vi "Programmingapplication_429B.vi"() -> (0 "command line":string=" -openD:\\20161122\\LNK01E-213300ALF\\LNK213-300ALF\\SW0077076V1-04.hex", 3 "Result":bool)   [LabVIEW 2011]
panel:
  out "text":string
  out "match + rest of string":string
  out "standard output":string
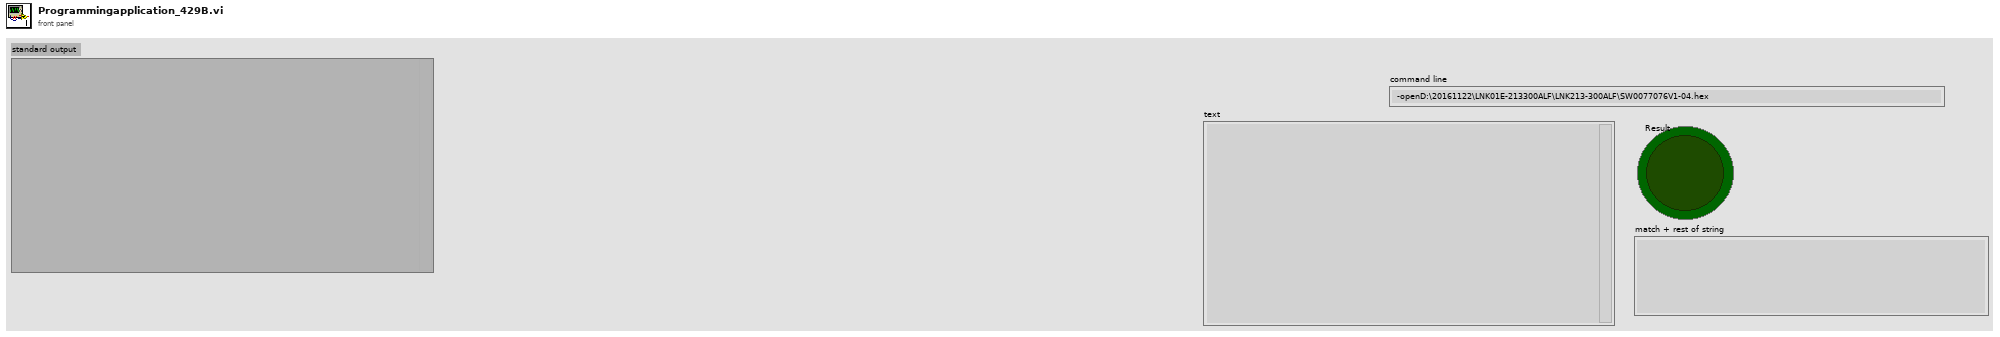
[diagram p1: front panel]
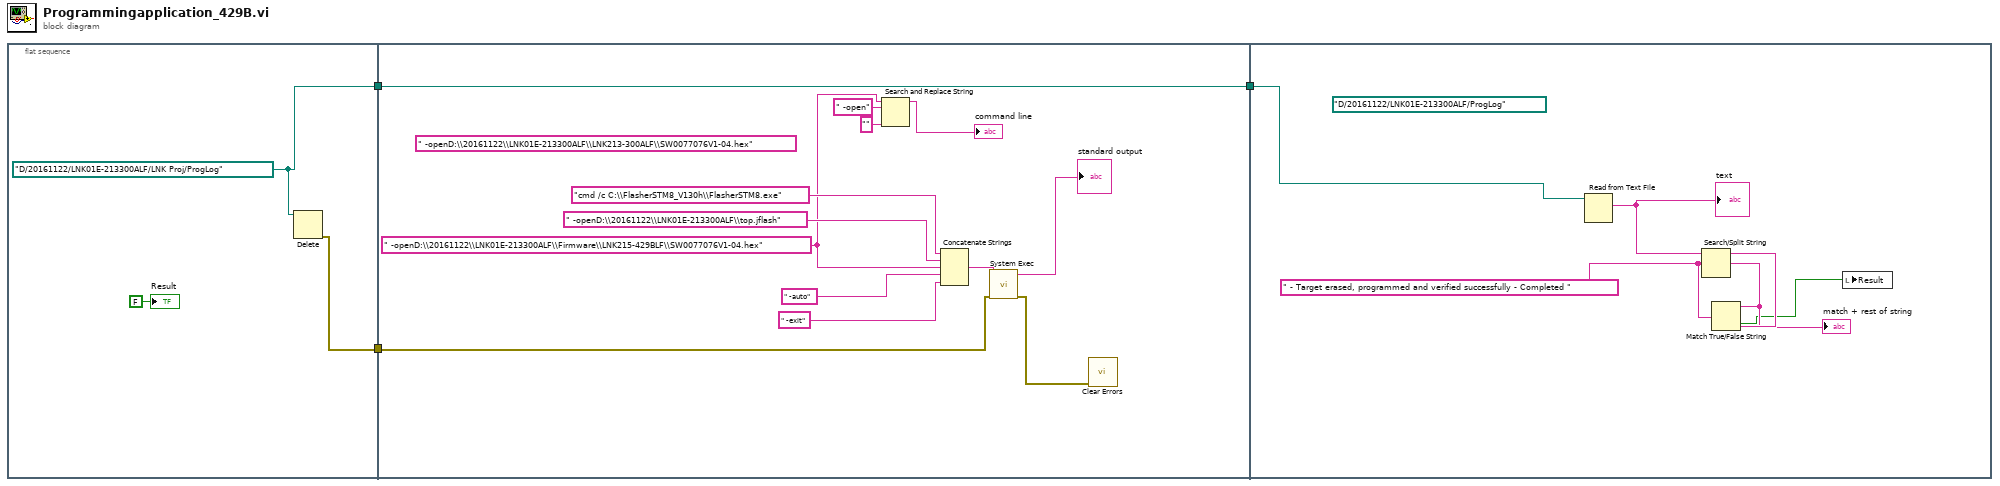
[diagram p0: block diagram]
diagram:
  n1 = flat-sequence {
    tunnel: [w6] -> w3
    tunnel: [w4] -> w1
    tunnel: w3 -> [w14]
    tunnel: [w7] -> w2
    tunnel: w1 -> [w7]
    tunnel: w2 -> [w20]
    frame #0 {
      w4 = path "D:/20161122/LNK01E-213300ALF/LNK Proj/ProgLog" ("file (use dialog)")
      n2 = Delete(path (use dialog)=w4) -> (error out=w6:errorcluster)  [unwired: 4 in, 2 out]
      "Result" <- FALSE ("Result")
    }
    frame #1 {
      (unwired) " -openD:\\20161122\\LNK01E-213300ALF\\LNK213-300ALF\\SW0077076V1-04.hex" ("command line")
      w11 = " -openD:\\20161122\\LNK01E-213300ALF\\Firmware\\LNK215-429BLF\\SW0077076V1-04.hex" ("command line")
      n3 = Search and Replace String(input string=w11, search string=" -open", replace string="" ("replace string (\"\")")) -> (result string=→"command line":string)  [unwired: 5 in, 3 out]
      n4 = Concatenate Strings("cmd /c C:\\FlasherSTM8_V130h\\FlasherSTM8.exe" ("command line"), " -openD:\\20161122\\LNK01E-213300ALF\\top.jflash" ("command line"), w11, " -auto" ("string"), " -exit" ("command line")) -> (w18:string)
      n5 = call <vilib>:"System Exec.vi"("error in (no error)"=w14, "command line"=w18) -> ("error out"=w19:errorcluster, "standard output"=→"standard output":string)  [unwired: 6 in, 2 out]
      n6 = call <vilib>:"Clear Errors.vi"("error in (no error)"=w19) -> ()  [unwired: 5 in, 2 out]
    }
    frame #2 {
      w23 = " - Target erased, programmed and verified successfully - Completed " ("search string/char (-)")
      (unwired) path "D:/20161122/LNK01E-213300ALF/ProgLog" ("file (use dialog)")
      n7 = Read from Text File(file (use dialog)=w20) -> (text=w22:string)  [unwired: 3 in, 3 out]
      "text" <- w22
      n8 = Search/Split String(string=w22, search string/char (-)=w23) -> (substring before match=w25:string, match + rest of string=w24:string)  [unwired: 1 in, 1 out]
      "match + rest of string" <- w24
      n9 = Match True/False String(2:w25, 3:w23, 4:w24) -> (0:w21:bool)  [unwired: 1 out]
      n10 = local write "Result"(w21) -> ()
    }
  }
